vi "Initialize Menu Items.vi"(8 "error in (no error)":errorcluster, 10 "Config":T1, 11 "Menu Ref":refnum<k9>) -> (0 "error out":errorcluster)   [LabVIEW 2023, in "VI Properties Editor.lvlib"]
doc: "Initializes several menu items related to options and recently viewed folders/files in <B>Config</B>."
uses:
  VI Properties Editor.lvlib
  CTLs/Config.ctl
  CTLs/Column Name.ctl
  CTLs/Filter Type.ctl
  CTLs/Filter Info.ctl
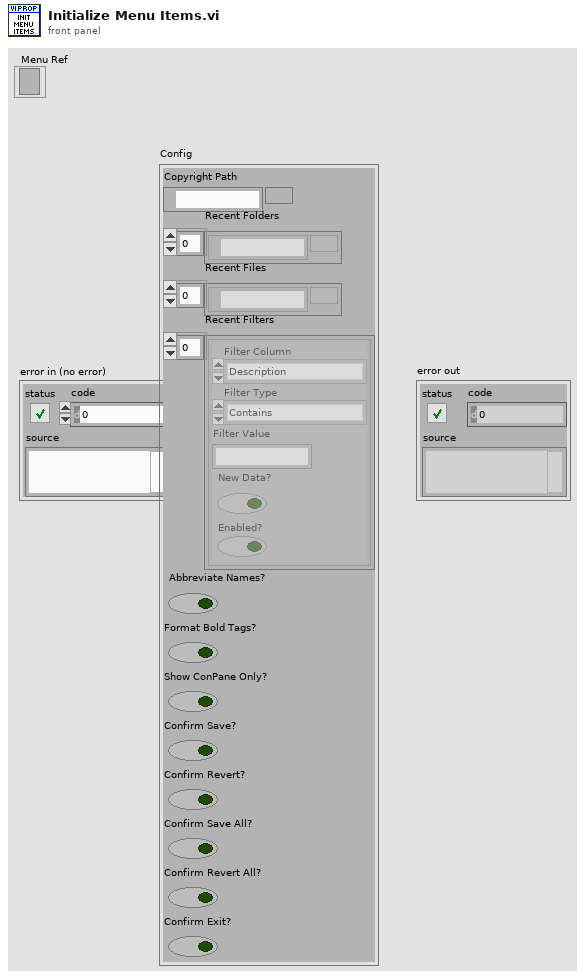
[diagram p1: front panel]
types:
  T1 = typedef "VI Properties Editor.lvlib/Config.ctl" = cluster{"Copyright Path":path, "Recent Folders":path[], "Recent Files":path[], "Recent Filters":T2[], "Abbreviate Names?":bool, "Format Bold Tags?":bool, "Show ConPane Only?":bool, "Confirm Save?":bool, "Confirm Revert?":bool, "Confirm Save All?":bool, "Confirm Revert All?":bool, "Confirm Exit?":bool}
  T2 = typedef "VI Properties Editor.lvlib/Filter Info.ctl" = cluster{"Filter Column":T3, "Filter Type":T4, "Filter Value":string, "New Data?":bool, "Enabled?":bool}
  T3 = typedef "VI Properties Editor.lvlib/Column Name.ctl" = enum16{"Name", "Path", "Type", "Window Title", "Description", "Help Path", "Help Tag", "Custom Title?", "Reentrant?", "Inlined?"}
  T4 = typedef "VI Properties Editor.lvlib/Filter Type.ctl" = enum16{"Contains", "Equals", "Starts with", "Ends with", "Does not contain", "Does not equal", "Is empty", "Is not empty"}
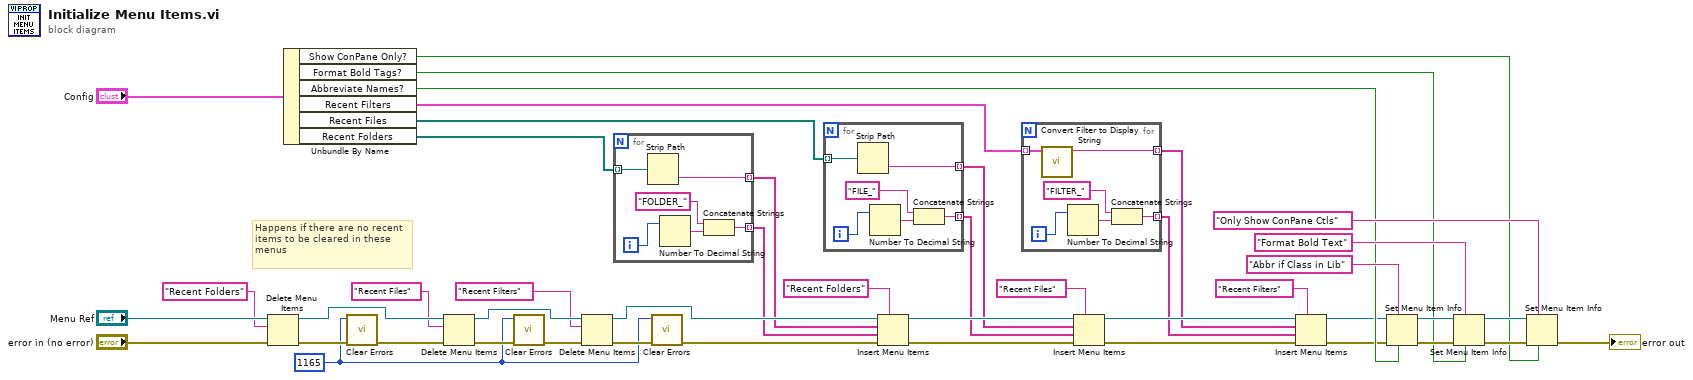
[diagram p0: block diagram]
diagram:
  w1 = 1165
  # "Happens if there are no recent items to be cleared in these menus"
  n1 = Delete Menu Items(6:"error in (no error)", 8:"Recent Folders" ("menu tag"), 9:"Menu Ref") -> (0:w21:errorcluster, 3:w43:refnum<k9>)  [unwired: 1 in]
  n2 = Unbundle By Name("Config") -> ("Show ConPane Only?"=w13:bool, "Format Bold Tags?"=w23:bool, "Abbreviate Names?"=w24:bool, "Recent Filters"=w12:T2[], "Recent Files"=w27:path[], "Recent Folders"=w33:path[])
  n3 = call <vilib>:"Clear Errors.vi"("error in (no error)"=w21, "specific error code to clear (0: all)"=w1) -> ("error out"=w16:errorcluster)  [unwired: 4 in, 1 out]
  n4 = Delete Menu Items(6:w16, 8:"Recent Files" ("menu tag"), 9:w43) -> (0:w22:errorcluster, 3:w4:refnum<k9>)  [unwired: 1 in]
  n5 = call <vilib>:"Clear Errors.vi"("error in (no error)"=w22, "specific error code to clear (0: all)"=w1) -> ("error out"=w17:errorcluster)  [unwired: 4 in, 1 out]
  n6 = Delete Menu Items(6:w17, 8:"Recent Filters" ("menu tag"), 9:w4) -> (0:w5:errorcluster, 3:w45:refnum<k9>)  [unwired: 1 in]
  n7 = for {
    tunnel: w33 -> [w50] mode=indexing
    tunnel: [w47] -> w28 mode=indexing
    tunnel: [w46] -> w29 mode=indexing
    i -> [w51]
    n8 = Strip Path(path=w50) -> (name=w46:string)  [unwired: 1 out]
    n9 = Number To Decimal String(number=w51) -> (decimal integer string=w49:string)  [unwired: 1 in]
    n10 = Concatenate Strings("FOLDER_", w49) -> (w47:string)
  }
  n11 = call <vilib>:"Clear Errors.vi"("error in (no error)"=w5, "specific error code to clear (0: all)"=w1) -> ("error out"=w2:errorcluster)  [unwired: 4 in, 1 out]
  n12 = for {
    tunnel: w27 -> [w56] mode=indexing
    tunnel: [w53] -> w26 mode=indexing
    tunnel: [w52] -> w25 mode=indexing
    i -> [w57]
    n13 = Strip Path(path=w56) -> (name=w52:string)  [unwired: 1 out]
    n14 = Number To Decimal String(number=w57) -> (decimal integer string=w55:string)  [unwired: 1 in]
    n15 = Concatenate Strings("FILE_", w55) -> (w53:string)
  }
  n16 = Insert Menu Items(5:"Recent Folders" ("menu tag"), 6:w2, 7:w28, 8:w29, 9:w45) -> (0:w39:errorcluster, 3:w30:refnum<k9>)  [unwired: 1 in, 1 out]
  n17 = for {
    tunnel: [w60] -> w7 mode=indexing
    tunnel: w12 -> [w59] mode=indexing
    tunnel: [w58] -> w6 mode=indexing
    i -> [w63]
    n18 = call "Convert Filter to Display String.vi"("Filter Info"=w59) -> ("String"=w58:string)  [unwired: 10 in]
    n19 = Number To Decimal String(number=w63) -> (decimal integer string=w62:string)  [unwired: 1 in]
    n20 = Concatenate Strings("FILTER_", w62) -> (w60:string)
  }
  n21 = Insert Menu Items(5:"Recent Files" ("menu tag"), 6:w39, 7:w26, 8:w25, 9:w30) -> (0:w38:errorcluster, 3:w10:refnum<k9>)  [unwired: 1 in, 1 out]
  n22 = Insert Menu Items(5:"Recent Filters" ("menu tag"), 6:w38, 7:w7, 8:w6, 9:w10) -> (0:w11:errorcluster, 3:w9:refnum<k9>)  [unwired: 1 in, 1 out]
  n23 = Set Menu Item Info(6:w24, 7:"Abbr if Class in Lib" ("menu tag"), 8:w11, 11:w9) -> (0:w42:errorcluster, 3:w35:refnum<k9>)  [unwired: 3 in]
  n24 = Set Menu Item Info(6:w23, 7:"Format Bold Text" ("item tag"), 8:w42, 11:w35) -> (0:w41:errorcluster, 3:w14:refnum<k9>)  [unwired: 3 in]
  n25 = Set Menu Item Info(6:w13, 7:"Only Show ConPane Ctls" ("item tag"), 8:w41, 11:w14) -> (0:→"error out":errorcluster)  [unwired: 3 in, 1 out]
